vi "KiberoUnpackToBinary.vi"(0 "Choose Directory":path) -> ()   [LabVIEW 2022 SP3]
uses:
  RF Data Value Reference.ctl
  Data Record.ctl
panel:
  out "Acoustic Data":T1
  out "Image Data":dbl[][](array[numeric])
  out "data values":T2
  in  "file ext":string="*"
  in  "Use Selected Files":bool
  in  "Listbox":i32[](listbox)
  # "Directoy of data"
  # "Kibero raw files have no extension"
  # "Select the kibero files. They will be resaved as a .dat file"
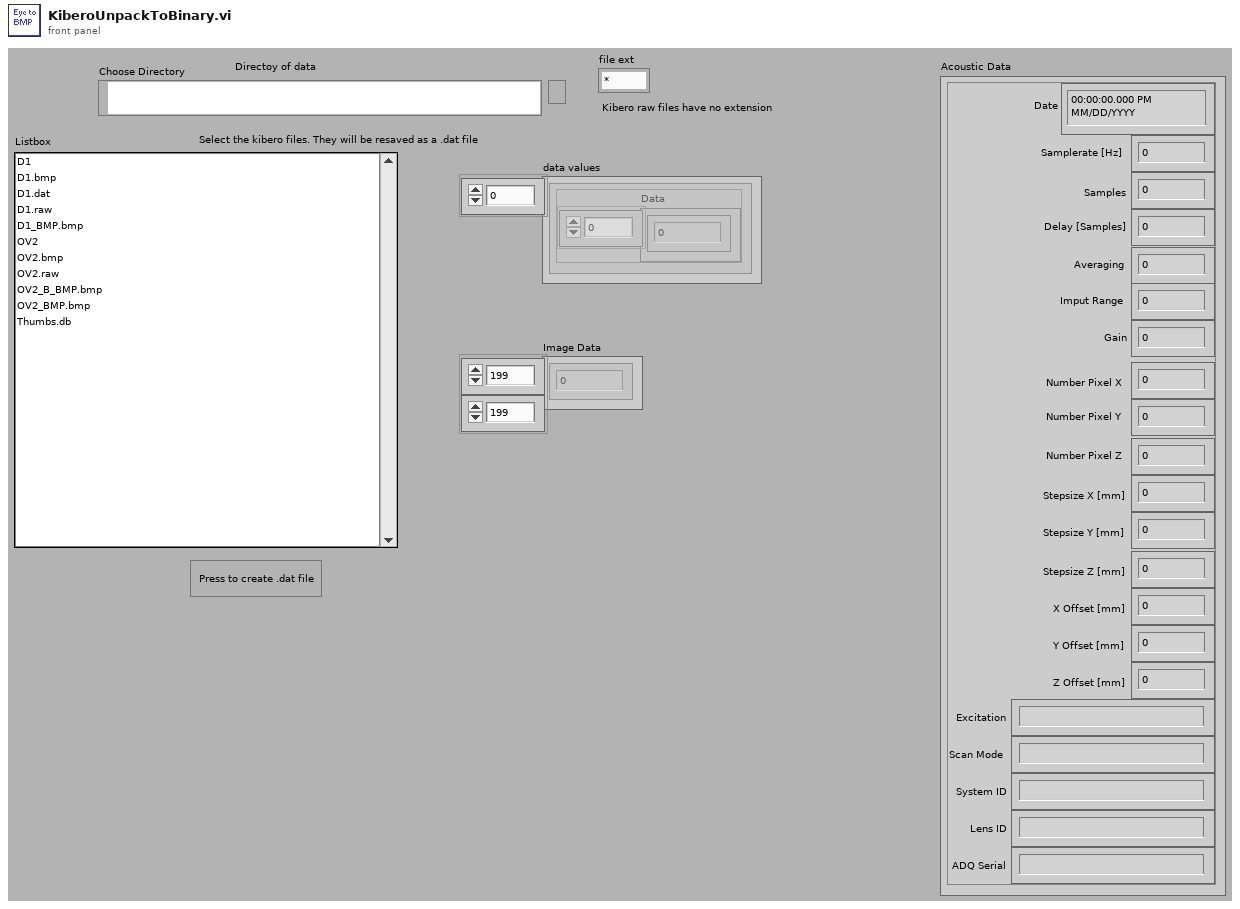
[diagram p1: front panel]
types:
  T1 = typedef "Data Record.ctl" = cluster{"Samplerate [Hz] ":dbl, "Delay [Samples]":i32, "Stepsize X [mm]":dbl, "Stepsize Y [mm]":dbl, "Z Offset [mm]":dbl, "Number Pixel X":i32, "Samples":i32, "Number Pixel Y":i32, "System ID":string, "Lens ID":string, "Date":timestamp, "X Offset [mm]":dbl, "Y Offset [mm]":dbl, "Scan Mode":string, "Excitation":string, "Gain":dbl, "Imput Range":dbl, "Averaging":i32, "ADQ Serial":string, "Stepsize Z [mm]":dbl, "Number Pixel Z":i32}
  T2 = typedef "RF Data Value Reference.ctl" = cluster{"Data":sgl[]}[]
  T3 = enum16{"open", "replace", "create", "open or create", "replace or create", "replace or create with confirmation"}
  T4 = enum16{"big-endian, network order", "native, host order", "little-endian"}
  T5 = typedef "Header.ctl" = cluster{"header info":cluster{"Header":string, "Head length":i16}, "A/D info":cluster{"# rf points per line":u16, "# lines per scan":u16, "sample rate MHz":u16, "# A/D bits":i16, "# bytes per A/D":u16, "TGC Flag":u16, "A/D Type":string}, "Tranducer Info":cluster{"bandwidth":sgl, "center freq":sgl, "start freq":sgl, "ID":i32}, "Scan Info":cluster{"delay":sgl, "pivot distance":sgl, "sector scan angle":sgl, "operator":string, "Scan Mode":string, "location":string}, "Time/Date Info":cluster{"date":string, "time":string}, "RF Info":cluster{"RF file name":string, "RF file att":string, "RF cal file name":string, "RF cal file att":string}, "Patient Info":cluster{"ID":string, "extended ID":string, "age":u16, "sex":string, "previously\nscanned":string, "PSA":sgl, "LOS":u8, "Ethnicty 2":u8, "Race":u8}, "Tissue Type":cluster{"organ":i16, "disease type":i16, "disease location":i16, "IQ_pts":u16, "RcvBuffer":u8, "RcvFrame":u16, "IQBuff":u8, "IQFrame":u16, "IQPage":u8}, "Votage scaling":cluster{"Digitizer (dB)":sgl, "Gain (dB)":sgl, "Atten (dB)":sgl}, "Comment":string, "Misc Info":cluster{"avg num":u16, "c speed":i16, "Div By or SF zones":i16, "XMIT CHS":u8, "RCV CHS":u8, "Xmit angle":sgl}, "Therapy Parameters":cluster{"Theraputic Freq (MHz)":sgl, "Time on (s)":sgl, "Therapy amplitude (mV)":sgl, "Lines Before":u16, "Lines After":u16}, "Scan Settings":cluster{"Energy (uJ or V)":u8, "Damp (Ohm) or Fc":u8, "HP Filt (KHz)":u8, "LP Filt (MHz)":u8, "Gain (db)":u8, "prf (kHz)":sgl, "Distance between\nscan lines (um)":u16, "Distance between\nscan planes (um)":u16, "Scan line gap (um)":sgl, "Scan plane gap (um)":sgl}, "Compression Parameters":cluster{"F1 (MHz)":sgl, "F2 (MHz)":sgl, "% taper":sgl, "duration":sgl}, "Patient Info Xtra":cluster{"First Name":string, "Last Name":string, "Notes":string}, "ROI Box":u16[]}
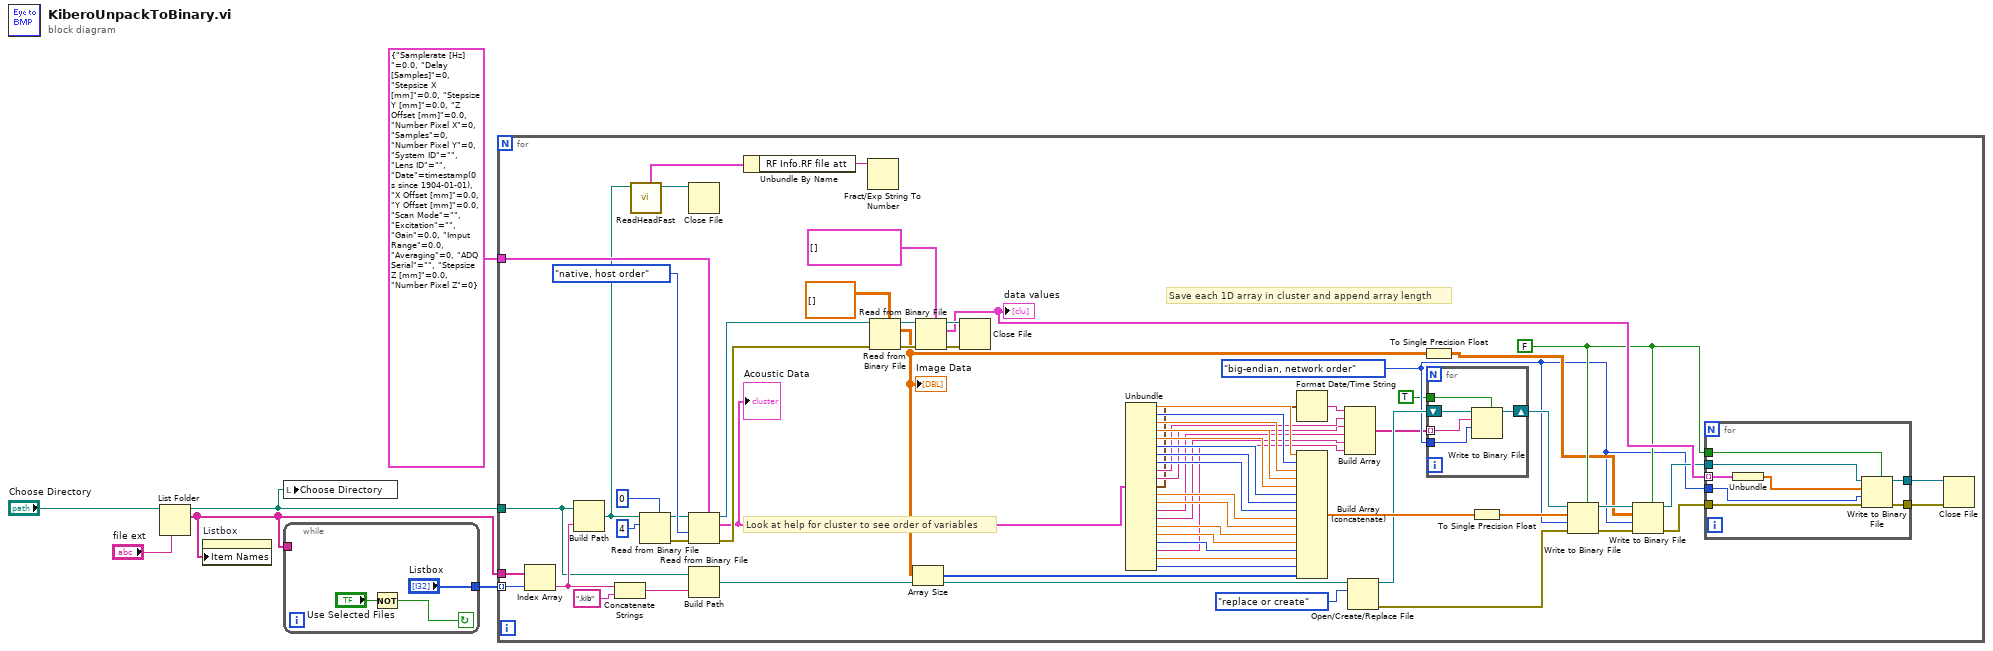
[diagram p0: block diagram]
diagram:
  n1 = List Folder(path="Choose Directory", pattern="file ext") -> (path out=w3:path, filenames=w6:string[])  [unwired: 1 in, 3 out]
  n2 = property on="Listbox" class="LstBox (strict)"("Item Names"=w6) -> ()  [unwired: 2 in, 2 out]
  n3 = local write "Choose Directory"(w3) -> ()
  n4 = while {
    tunnel: ["Listbox"] -> w5
    tunnel: w6 -> [_]
    stop <- w9 continue-if-true
    n5 = Not(x="Use Selected Files") -> (.not. x?=w9:bool)
  }
  n6 = for {
    tunnel: w6 -> [w76]
    tunnel: w5 -> [w75] mode=indexing
    tunnel: w3 -> [w31]
    tunnel: T1 {"Samplerate [Hz] "=0.0, "Delay [Samples]"=0, "Stepsize X [mm]"=0.0, "Stepsize Y [mm]"=0.0, "Z Offset [mm]"=0.0, "Number Pixel X"=0, "Samples"=0, "Number Pixel Y"=0, "System ID"="", "Lens ID"="", "Date"=timestamp(0 s since 1904-01-01), "X Offset [mm]"=0.0, "Y Offset [mm]"=0.0, "Scan Mode"="", "Excitation"="", "Gain"=0.0, "Imput Range"=0.0, "Averaging"=0, "ADQ Serial"="", "Stepsize Z [mm]"=0.0, "Number Pixel Z"=0} ("Acoustic Data") -> [w63]
    w14 = T4."big-endian, network order" ("byte order (0:big-endian, network order)")
    w27 = FALSE ("prepend array or string size? (T)")
    # "Look at help for cluster to see order of variables"
    # "Save image data with dimensions appenended"
    # "Save each 1D array in cluster and append array length"
    n7 = Index Array(array=w76, index=w75) -> (element=w42:string)
    n8 = Build Path(base path=w31, name or relative path=w42) -> (appended path=w40:path)
    n9 = Concatenate Strings(w42, ".kib") -> (w39:string)
    n10 = call "ReadHeadFast.vi"("new file path"=w40) -> ("refnum out"=w73:refnum<file>, "Header In"=w74:T5)  [unwired: 7 in, 2 out]
    n11 = Read from Binary File(5:u8 0, 10:4 ("count (1)"), 11:w40) -> (0:w59:errorcluster, 3:w60:refnum<file>)  [unwired: 3 in, 2 out]
    n12 = Close File(refnum=w73) -> ()  [unwired: 1 in, 2 out]
    n13 = Read from Binary File(5:w63, 8:w59, 9:T4."native, host order" ("byte order (0:big-endian, network order)"), 11:w60) -> (0:w68:errorcluster, 2:w58:T1, 3:w65:refnum<file>)  [unwired: 2 in, 1 out]
    "Acoustic Data" <- w58
    n14 = Build Path(base path=w31, name or relative path=w39) -> (appended path=w10:path)
    n15 = Unbundle By Name(w74) -> ("RF Info.RF file att"=w77:string)
    n16 = Fract/Exp String To Number(string=w77) -> ()  [unwired: 5 out]
    n17 = Read from Binary File(5:dbl[][] [], 8:w68, 11:w65) -> (0:w67:errorcluster, 2:w35:dbl[][], 3:w64:refnum<file>)  [unwired: 3 in, 1 out]
    "Image Data" <- w35
    n18 = Array Size(array=w35) -> (size(s)=w34:i32[])
    n19 = Read from Binary File(5:T2 [] ("Data Referenzen"), 8:w67, 11:w64) -> (0:w69:errorcluster, 2:w30:T2, 3:w70:refnum<file>)  [unwired: 3 in, 1 out]
    "data values" <- w30
    n20 = Close File(refnum=w70, error in=w69) -> ()  [unwired: 2 out]
    n21 = Unbundle(w58) -> ("Samplerate [Hz]"=w57:dbl, "Delay [Samples]"=w56:i32, "Stepsize X [mm]"=w55:dbl, "Stepsize Y [mm]"=w54:dbl, "Z Offset [mm]"=w53:dbl, "Number Pixel X"=w52:i32, "Samples"=w51:i32, "Number Pixel Y"=w50:i32, "System ID"=w22:string, "Lens ID"=w21:string, "Date"=w17:timestamp, "X Offset [mm]"=w49:dbl, "Y Offset [mm]"=w48:dbl, "Scan Mode"=w20:string, "Excitation"=w19:string, "Gain"=w47:dbl, "Imput Range"=w46:dbl, "Averaging"=w45:i32, "ADQ Serial"=w18:string, "Stepsize Z [mm]"=w44:dbl, "Number Pixel Z"=w43:i32)
    n22 = Format Date/Time String(seconds (now)=w17) -> (date/time string=w12:string)  [unwired: 2 in]
    n23 = Build Array (concatenate)(w57, w56, w55, w54, w53, w52, w51, w50, w49, w48, w47, w46, w45, w44, w43, w34) -> (w38:dbl[])
    n24 = Build Array(w12, w22, w21, w20, w19, w18) -> (w11:string[])
    n25 = Open/Create/Replace File(file path (use dialog)=w10, operation (0:open)=T3."replace or create") -> (refnum out=w16:refnum<file>, error out=w33:errorcluster)  [unwired: 4 in, 1 out]
    n26 = To Single Precision Float(number=w35) -> (single precision float=w23:sgl[][])
    n27 = for {
      tunnel: w14 -> [w80]
      tunnel: TRUE ("prepend array or string size? (T)") -> [w79]
      tunnel: w11 -> [w78] mode=indexing
      shift-right: [w81] -> w15
      shift-left: w16 -> [w82]
      n28 = Write to Binary File(file (use dialog)=w82, data=w78, 5:w79, 9:w80) -> (refnum out=w81:refnum<file>)  [unwired: 2 in, 2 out]
    }
    n29 = To Single Precision Float(number=w38) -> (single precision float=w24:sgl[])
    n30 = Write to Binary File(file (use dialog)=w15, data=w24, error in=w33, 5:w27, 9:w14) -> (refnum out=w37:refnum<file>, error out=w36:errorcluster)  [unwired: 1 in, 1 out]
    n31 = Write to Binary File(file (use dialog)=w37, data=w23, error in=w36, 5:w27, 9:w14) -> (refnum out=w29:refnum<file>, error out=w28:errorcluster)  [unwired: 1 in, 1 out]
    n32 = for {
      tunnel: w30 -> [w88] mode=indexing
      tunnel: w29 -> [w90]
      tunnel: w28 -> [w89]
      tunnel: w27 -> [w87]
      tunnel: [w86] -> w26
      tunnel: [w85] -> w25
      tunnel: w14 -> [w84]
      n33 = Unbundle(w88) -> ("Data"=w83:sgl[])
      n34 = Write to Binary File(file (use dialog)=w90, data=w83, error in=w89, 5:w87, 9:w84) -> (refnum out=w86:refnum<file>, error out=w85:errorcluster)  [unwired: 1 in, 1 out]
    }
    n35 = Close File(refnum=w26, error in=w25) -> ()  [unwired: 2 out]
  }
